vi "Boolean Timer (Event) LV2012 NIVerified.vi"() -> ()   [LabVIEW 2018]
doc: "Demonstrates how to program a boolean timer ('stop watch') with events"
uses:
  <vilib>/Utility/file.llb/Write Delimited Spreadsheet (string).vi
panel:
  in  "stop":bool
  out "Time Difference (s)":dbl format="%.3f"
  in  "Start Stop Button":bool
  out "Current Timer (s)":dbl format="%.3f"
  # "Overview: Demonstrates how to program a boolean timer ('stop watch') with events\nRequirements: LabVIEW 2012 Base Development System (or compatible)\nInstructions: \n1. Run the VI\n2. Click the Start Watch Button to start the timer\n3. The Current Timer indicator updates every 10 ms\n4. Click the same button again to stop the timer\n5. The time difference is displayed and the timer stops updating"
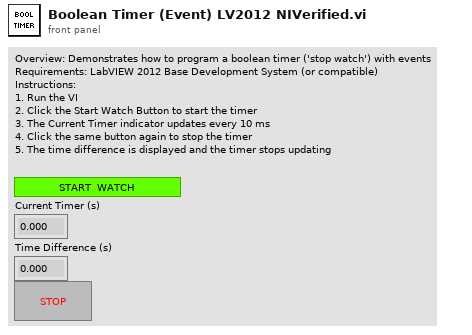
[diagram p1: front panel]
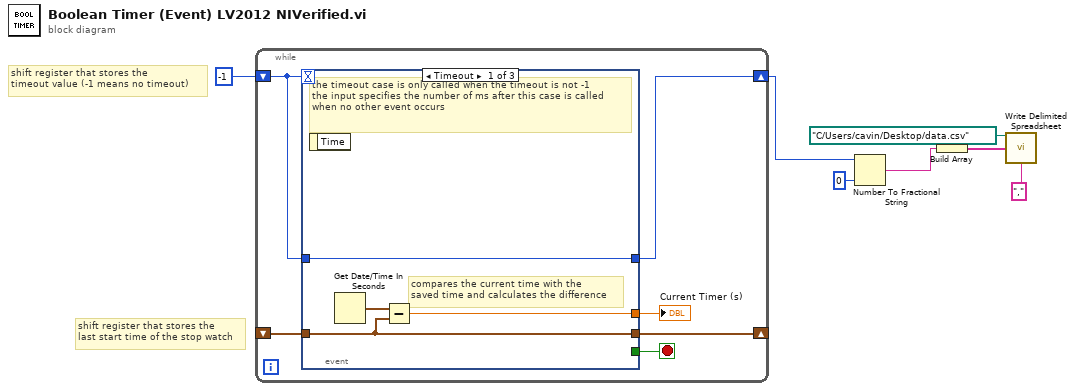
[diagram p0: block diagram]
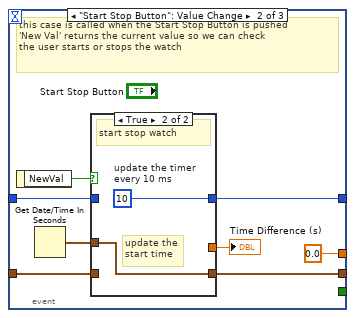
[diagram p2: hidden frame]
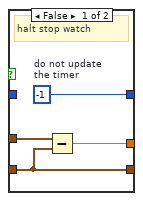
[diagram p3: hidden frame]
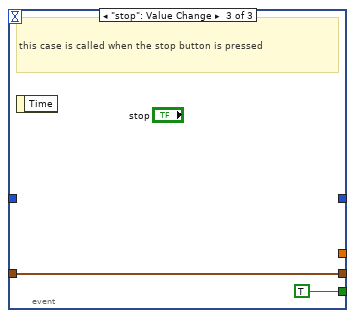
[diagram p4: hidden frame]
diagram:
  # "shift register that stores the\ntimeout value (-1 means no timeout)"
  # "shift register that stores the\nlast start time of the stop watch"
  n1 = while {
    shift-right: [w12] -> _
    shift-left: _ -> [w13]
    shift-right: [w9] -> w6
    shift-left: -1 -> [w10]
    stop <- w11 stop-if-true
    n2 = event shown="[0] Timeout" {
      selector: _ -> [_ _ _]
      dyn-events: _ -> [_ _ _]
      timeout: w10 -> [_ _ _]
      tunnel: w13 -> [w16 w23 w32]
      tunnel: [w16 w24 w32] -> w12
      tunnel: [_ _ TRUE] -> w11
      tunnel: w10 -> [w15 w21 _]
      tunnel: [w15 w20 _] -> w9
      tunnel: [w14 0.0 _] -> w8
      event Timeout {
        # "compares the current time with the\nsaved time and calculates the difference"
        # "the timeout case is only called when the timeout is not -1\nthe input specifies the number of ms after this case is called\nwhen no other event occurs"
        n3 = event-data() -> ()  [unwired: 1 in, 1 out]
        n4 = Get Date/Time In Seconds() -> (seconds since 1Jan1904=w17:timestamp)
        n5 = Subtract(x=w17, y=w16) -> (x-y=w14:dbl)
      }
      event "Start Stop Button": Value Change {
        # "this case is called when the Start Stop Button is pushed\n'New Val' returns the current value so we can check\nthe user starts or stops the watch"
        n6 = event-data() -> ("NewVal"=w25:bool)  [unwired: 1 in]
        n7 = Get Date/Time In Seconds() -> (seconds since 1Jan1904=w22:timestamp)
        n8 = case shown="True" w25 {
          tunnel: [w29 w31] -> w24
          tunnel: w23 -> [w29 _]
          tunnel: w22 -> [w28 w31]
          tunnel: w21 -> [_ _]
          tunnel: [w27 w30] -> w20
          tunnel: [w26 _] -> w19
          frame False {
            w27 = -1  # do not update the timer
            # "halt stop watch"
            n9 = Subtract(x=w28, y=w29) -> (x-y=w26:dbl)
          }
          frame True {
            w30 = 10  # update the timer every 10 ms
            # "update the\nstart time"
            # "start stop watch"
          }
        }
        "Time Difference (s)" <- w19
      }
      event "stop": Value Change {
        # "this case is called when the stop button is pressed"
        n10 = event-data() -> ()  [unwired: 1 in, 1 out]
      }
    }
    "Current Timer (s)" <- w8
  }
  n11 = Number To Fractional String(number=w6, precision (6)=i16 0) -> (F-format string=w4:string)  [unwired: 2 in]
  n12 = Build Array(w4) -> (w3:string[])
  n13 = call-poly <vilib>:"Write Delimited Spreadsheet.vi"("file path (dialog if empty)"=path "C:/Users/cavin/Desktop/data.csv", "1D data"=w3, "delimiter (\\t)"="," ("delimiter (\\t)")) -> ()  [unwired: 11 in, 2 out]
